vi "Creator Queue.vi"(9 "Priority?":bool, 10 "Msg Strategy":refnum<class "Msg Strategy.lvclass">, 11 "Base Queue in":refnum<class "Base Queue.lvclass">) -> (3 "Base Queue out":refnum<class "Base Queue.lvclass">)   [LabVIEW 2021, in "jettl.lvlib" / "Base Queue.lvlib" / "Base Queue.lvclass"]
uses:
  Base Queue.lvclass
  Base Queue.lvclass/Base Queue.ctl
  Msg Strategy/Msg Strategy.lvclass
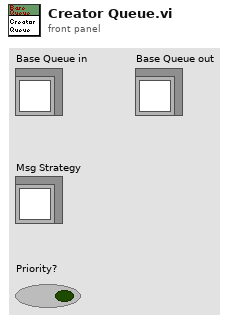
[diagram p1: front panel]
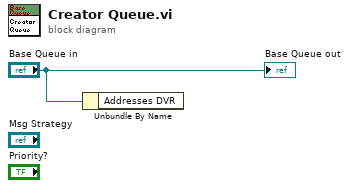
[diagram p0: block diagram]
diagram:
  n1 = Unbundle By Name("Base Queue in") -> ()  [unwired: 1 out]
  "Base Queue out" <- "Base Queue in"
